vi "Shutdown.vi"(8 "error in (no error)":errorcluster, 11 "DSFPlugin in":refnum<class "DSFPlugin Transceiver.lvclass">) -> (0 "error out":errorcluster, 3 "DSFPlugin out":refnum<class "DSFPlugin Transceiver.lvclass">)   [LabVIEW 2017, in "DSFPluginTest.lvlib" / "DSFPlugin Transceiver.lvclass"]
uses:
  DSFPlugin Transceiver.lvclass
  DSFPlugin Transceiver.lvclass/DSFPlugin Transceiver.ctl
  builds/Data Sharing Framework/Current/Data Sharing Framework Core/DSF Core.lvlibp/Engine/Classes/Transceiver/Transceiver.lvclass
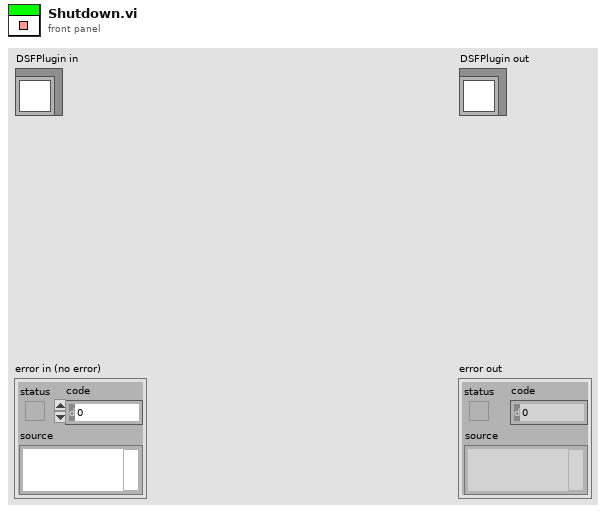
[diagram p1: front panel]
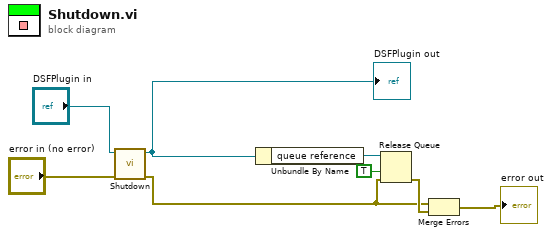
[diagram p0: block diagram]
diagram:
  n1 = call-parent "Shutdown.vi"("error in (no error)"="error in (no error)", "Transceiver in"="DSFPlugin in") -> ("error out"=w3:errorcluster, "Transceiver out"=w2:refnum<class "DSFPlugin Transceiver.lvclass">)  [unwired: 8 in]
  "DSFPlugin out" <- w2
  n2 = Unbundle By Name(w2) -> ("queue reference"=w6:refnum<queue>)
  n3 = Release Queue(queue=w6, force destroy? (F)=TRUE, error in (no error)=w3) -> (error out=w5:errorcluster)  [unwired: 2 out]
  n4 = Merge Errors(w3, w5) -> (→"error out":errorcluster)
